vi "State_Send_GPIO.vi"(7 "Mode":enum16{"User valves", "Auto valves"}(ring), 8 "User valves in":bool[](array[boolean]), 9 "Auto valves in":bool[][](array[boolean])) -> (3 "BBB command out":string)   [LabVIEW 2025]
uses:
  TypeDef_BBBJSON_commands.ctl
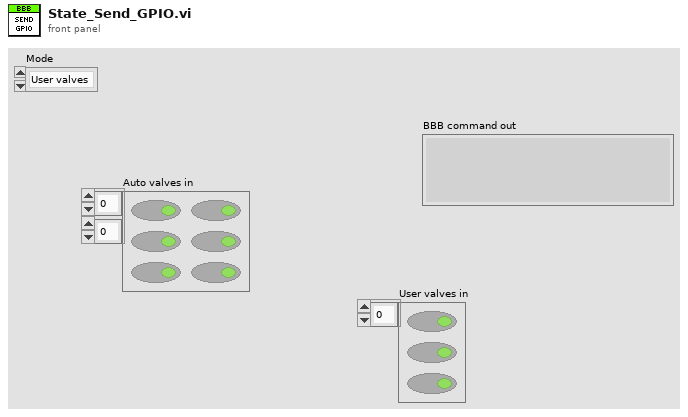
[diagram p1: front panel]
types:
  T1 = typedef "TypeDef_BBBJSON_commands.ctl" = cluster{"SetState":cluster{"StateNum":i32}, "SetSave":cluster{"Save":i16}, "SetTEC":cluster{"TargetT":dbl, "Reset":i32, "Enable":i32}, "SetMFC":cluster{"MFC0":dbl, "MFC1":dbl}, "SetGPIO":cluster{"SSR0":i16, "SSR1":i16, "LED":i16}}
  T2 = cluster{"SetGPIO":cluster{"SSR0":i16, "SSR1":i16, "LED":i16}}
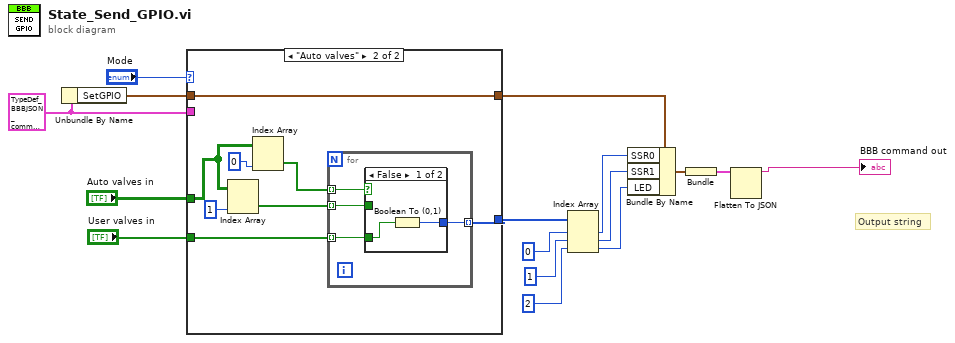
[diagram p0: block diagram]
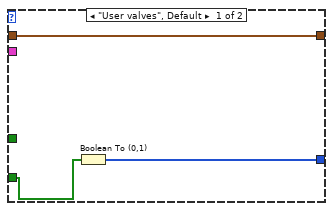
[diagram p2: hidden frame]
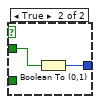
[diagram p3: hidden frame]
diagram:
  w13 = T1 {"SetState"={"StateNum"=0}, "SetSave"={"Save"=0}, "SetTEC"={"TargetT"=0.0, "Reset"=0, "Enable"=0}, "SetMFC"={"MFC0"=0.0, "MFC1"=0.0}, "SetGPIO"={"SSR0"=0, "SSR1"=0, "LED"=0}} ("BBBcommands")
  # "Output string"
  n1 = Unbundle By Name(w13) -> ("SetGPIO"=w3:cluster{"SSR0":i16, "SSR1":i16, "LED":i16})
  n2 = case shown="\"Auto valves\"" "Mode" {
    tunnel: "Auto valves in" -> [_ w25]
    tunnel: "User valves in" -> [w19 w22]
    tunnel: w13 -> [_ _]
    tunnel: [w18 w21] -> w10
    tunnel: w3 -> [w17 w20]
    tunnel: [w17 w20] -> w2
    frame "User valves", Default {
      n3 = Boolean To (0,1)(Boolean=w19) -> (0, 1=w18:i16[])
    }
    frame "Auto valves" {
      n4 = Index Array(array=w25, index (col)=1 ("disabled index (col)")) -> (element=w23:bool[])  [unwired: 1 in]
      n5 = Index Array(array=w25, index (col)=0 ("disabled index (col)")) -> (element=w24:bool[])  [unwired: 1 in]
      n6 = for {
        tunnel: w24 -> [w30] mode=indexing
        tunnel: w23 -> [w31] mode=indexing
        tunnel: w22 -> [w29] mode=indexing
        tunnel: [w28] -> w21 mode=indexing
        n7 = case shown="False" w30 {
          tunnel: w31 -> [_ w35]
          tunnel: w29 -> [w33 _]
          tunnel: [w32 w34] -> w28
          frame False {
            n8 = Boolean To (0,1)(Boolean=w33) -> (0, 1=w32:i16)
          }
          frame True {
            n9 = Boolean To (0,1)(Boolean=w35) -> (0, 1=w34:i16)
          }
        }
      }
    }
  }
  n10 = Index Array(array=w10, index #1=0 ("index"), index #2=1 ("index"), index #3=2 ("index")) -> (element #1=w6:i16, element #2=w5:i16, element #3=w4:i16)
  n11 = Bundle By Name(cluster=w2, "SSR0"=w6, "SSR1"=w5, "LED"=w4) -> (w11:cluster{"SSR0":i16, "SSR1":i16, "LED":i16})
  n12 = Bundle("SetGPIO"=w11) -> (w12:T2)  [unwired: 1 in]
  n13 = Flatten To JSON(anything=w12) -> (JSON string=→"BBB command out":string)  [unwired: 2 in, 1 out]
